vi "Proyecto_Malabot.vi"() -> ()   [LabVIEW 2019]
panel:
  in  "stop":bool
  out "Motor 2 sensor":dbl
  out "Motor 1 sensor":dbl
  in  "Señal_5 2":dbl
  in  "Power Motor griper":dbl
  in  "Set Motor 2":dbl
  in  "Set Motoro 1":dbl
  in  "Angulo Servo A":dbl
  out "Trama de envio 2":string
  out "TOF":dbl
  out "US 2":dbl
  out "US 1":dbl
  out "Trama Recibida 2":string
  out "Sensor 5":dbl
  out "Sensor 4":dbl
  in  "Señal 5":dbl
  in  "Señal 4":dbl
  in  "Señal_3":dbl
  in  "Señal_2":dbl
  in  "Señal_1":dbl
  out "Trama de envio":string
  out "Sensor_3":dbl
  out "Sensor_2":dbl
  out "Sensor_1":dbl
  out "Trama Recibida":string
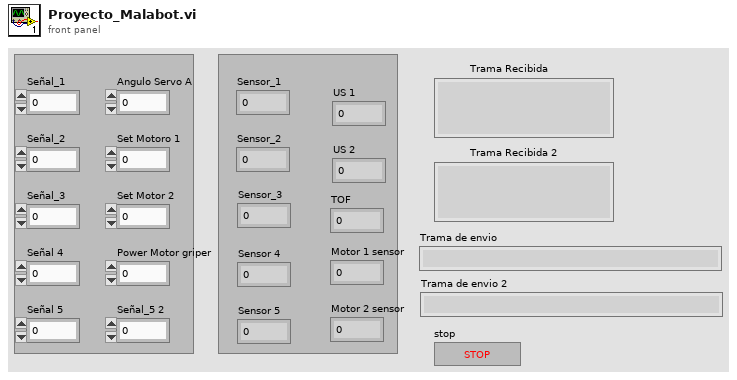
[diagram p1: front panel]
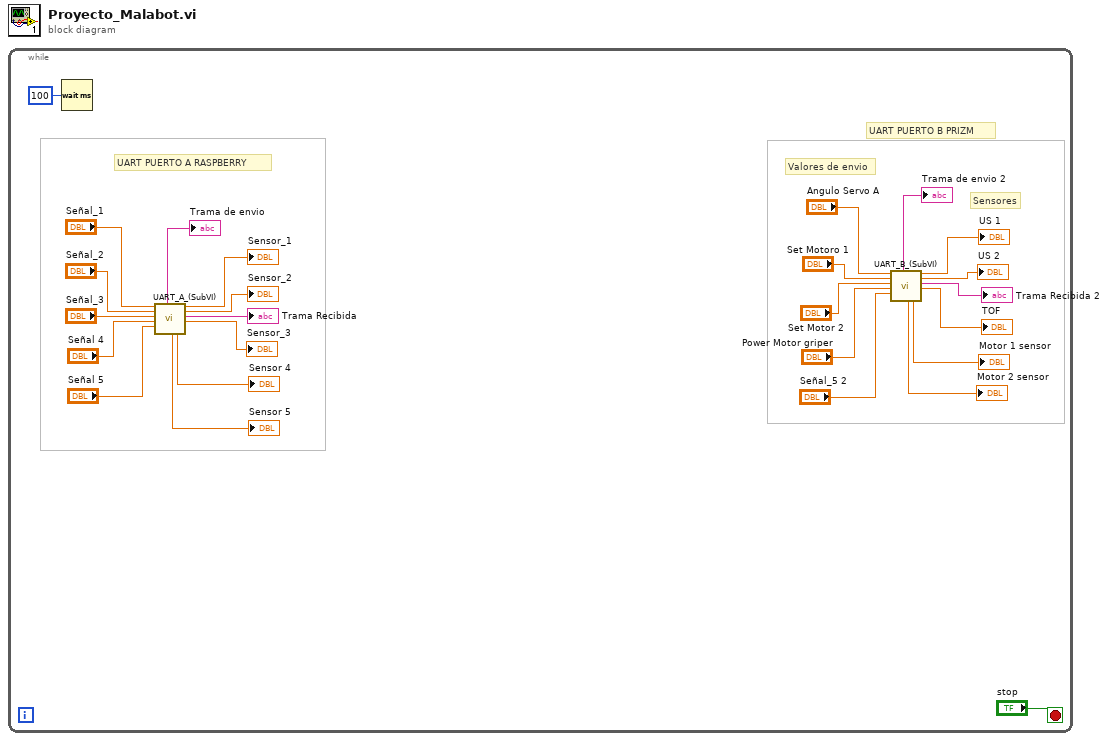
[diagram p0: block diagram]
diagram:
  n1 = while {
    stop <- "stop" stop-if-true
    # "Sensores"
    # "Valores de envio"
    # "UART PUERTO B PRIZM"
    # "UART PUERTO A RASPBERRY"
    n2 = Wait (ms)(milliseconds to wait=u32 100) -> ()  [unwired: 1 out]
    n3 = call "UART_A_(SubVI).vi"("Señal_1"="Señal_1", "Señal_2"="Señal_2", "Señal_3"="Señal_3", "Señal 4"="Señal 4", "Señal 5"="Señal 5") -> ("Trama de envio"=→"Trama de envio":string, "Sensor 5"=→"Sensor 5":dbl, "Sensor 4"=→"Sensor 4":dbl, "Sensor_1"=→"Sensor_1":dbl, "Sensor_2"=→"Sensor_2":dbl, "Trama Recibida"=→"Trama Recibida":string, "Sensor_3"=→"Sensor_3":dbl)  [unwired: 3 in, 5 out]
    n4 = call "UART_B_(SubVI).vi"("Señal_1 in"="Angulo Servo A", "Señal_2 in"="Set Motoro 1", "Señal_3 in"="Set Motor 2", "Señal 6"="Power Motor griper", "Señal 7"="Señal_5 2") -> ("Trama de envio 2"=→"Trama de envio 2":string, "Sensor 7"=→"Motor 2 sensor":dbl, "Sensor 6"=→"Motor 1 sensor":dbl, "Sensor_1 2"=→"US 1":dbl, "Sensor_2 2"=→"US 2":dbl, "Trama Recibida 2"=→"Trama Recibida 2":string, "Sensor_3 2"=→"TOF":dbl)  [unwired: 3 in, 5 out]
  }
